vi "Teleop.vi"(10 "Match Info":T1={"Autonomous Elapsed Seconds"=0.0, "TeleOp Elapsed Seconds"=0.0, "Disabled Elapsed Seconds"=0.0, "Visited Autonomous"=FALSE, "Visited TeleOp"=FALSE, "Visited Disabled"=FALSE, "Autonomous Settings"={"Autonomous Style"=enum."Independent", "VI Refnum"=refnum}}, 11 "Call Context":T2) -> ()   [LabVIEW 2014]
doc: "This VI is called for each TeleOp packet received from the DS where the robot is not disabled. It is often used to read from the joysticks and update I/O or to update setpoints for timed control loops. It should complete and return within 20 milliseconds or it may miss DS packets."
uses:
  <vilib>/Rock Robotics/WPI/DriverStation/WPI_DriverStationDerivedRobotMode.ctl
  <vilib>/Rock Robotics/WPI/DriverStation/WPI_DriverStationMatch Info.ctl
  <vilib>/Rock Robotics/WPI/RobotDrive/WPI_RobotDriveGetSetRefNum.vi
  <vilib>/Rock Robotics/WPI/Joystick/WPI_JoystickGetSetRefNum.vi
  <vilib>/Rock Robotics/Network Tables/SD Write Boolean Array.vi
  <vilib>/Rock Robotics/Network Tables/SD Write Numeric Array.vi
  <vilib>/Rock Robotics/Network Tables/SD Read Boolean.vi
  <vilib>/Rock Robotics/Network Tables/SD Read Number.vi
  <vilib>/Rock Robotics/WPI/RobotDrive/WPI_RobotDriveMecanumDrive_Cartesian.vi
panel:
  out "Sample Slider 0":dbl(slide) scale=0.0..5.0
  out "Sample Boolean 1":bool
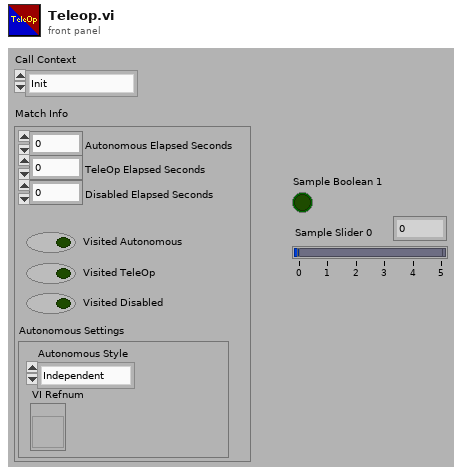
[diagram p1: front panel]
types:
  T1 = typedef "WPI_DriverStationMatch Info.ctl" = cluster{"Autonomous Elapsed Seconds":dbl, "TeleOp Elapsed Seconds":dbl, "Disabled Elapsed Seconds":dbl, "Visited Autonomous":bool, "Visited TeleOp":bool, "Visited Disabled":bool, "Autonomous Settings":cluster{"Autonomous Style":enum16{"Iterative", "Independent"}, "VI Refnum":refnum<vi>}}
  T2 = typedef "WPI_DriverStationDerivedRobotMode.ctl" = enum16{"Init", "Execute", "Stop"}
  T3 = typedef "WPI_JoystickDevRef.ctl" = cluster{"Device":T4}
  T4 = typedef "WPI_JoystickDeviceEnum.ctl" = enum16{"USB 0", "USB 1", "USB 2", "USB 3", "USB 4", "USB 5"}
  T5 = cluster{"Button 1":bool, "Button 2":bool, "Button 3":bool, "Button 4":bool, "Button 5":bool, "Button 6":bool, "Button 7":bool, "Button 8":bool, "Button 9":bool, "Button 10":bool, "Button 11":bool, "Button 12":bool}
  T6 = typedef "WPI_MotorControlDeviceRef.ctl" = cluster{"DeviceStatus":errorcluster, "Type":T7, "PWM":cluster{"Controller":T8, "PWM Channel":T9, "DeadBand":T10}, "CAN":cluster{"Device Number":u8, "Control Mode":T11, "Semaphore":T12, "Max Vout":dbl, "TalonSRX Control Mode":T13}, "Invert":bool, "TransformRef":T14, "InvTransformRef":T14}
  T7 = typedef "WPI_MotorControlType.ctl" = enum16{"PWM", "CAN", "CANTalonSRX"}
  T8 = typedef "FPGA_TypedefDigitalModule.ctl" = enum16{"Controller 1"}
  T9 = typedef "FPGA_DIOPWMChannel.ctl" = enum8{"PWM 0", "PWM 1", "PWM 2", "PWM 3", "PWM 4", "PWM 5", "PWM 6", "PWM 7", "PWM 8", "PWM 9", "PWM MXP 0", "PWM MXP 1", "PWM MXP 2", "PWM MXP 3", "PWM MXP 4", "PWM MXP 5", "PWM MXP 6", "PWM MXP 7", "PWM MXP 8", "PWM MXP 9", "Invalid"}
  T10 = typedef "WPI_PWMDeadband.ctl" = cluster{"Name":string, "maxPositivePwm":i32, "minPositivePwm":i32, "centerPwm":i32, "maxNegativePwm":i32, "minNegativePwm":i32, "angularRange":u16}
  T11 = typedef "WPI_CANJaguar_ControlMode.ctl" = enum8{"Percent VBus", "Current", "Speed", "Position", "Voltage"}
  T12 = typedef "Semaphore RefNum" = refnum<k1>
  T13 = typedef "WPI_CANTalonSRX_APIControlMode.ctl" = enum8{"Percent VBus", "Speed", "Position", "Slave", "Unchanged / Invalid"}
  T14 = typedef "WPI_PWMTransform_ConPane.ctl" = refnum<vi>
  T15 = typedef "WPI_RobotDriveDevRef.ctl" = cluster{"DevStatus":errorcluster, "Motors[]":T6[], "Square Inputs":bool, "Max Output":dbl}
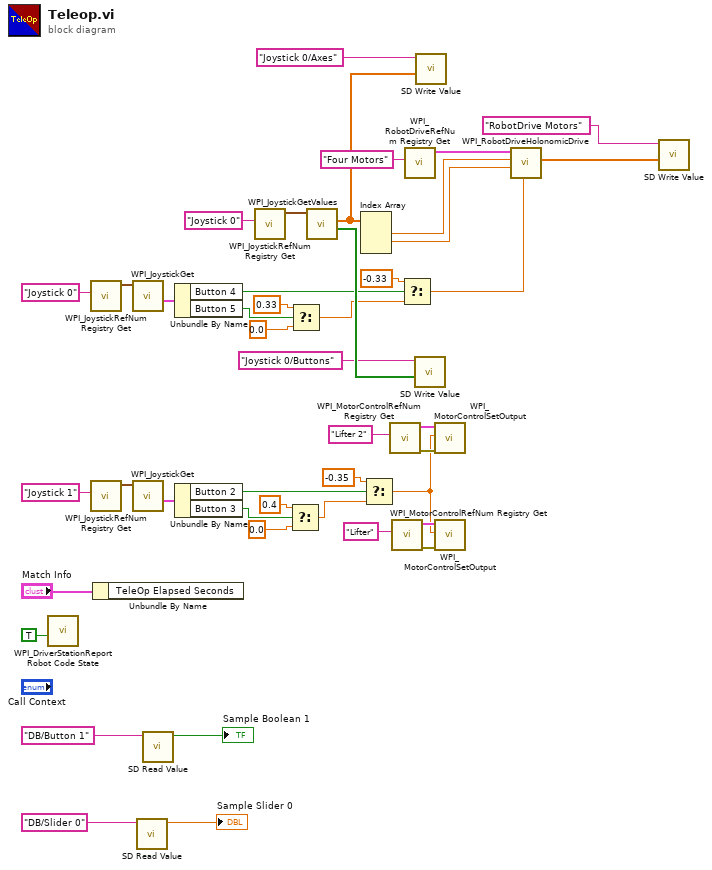
[diagram p0: block diagram]
diagram:
  n1 = call <vilib>:"WPI_DriverStationReport Robot Code State.vi"("TeleOp"=TRUE ("Autonomous")) -> ()  [unwired: 10 in, 1 out]
  n2 = call <vilib>:"WPI_JoystickRefNum Registry Get.vi"("refnum name"="Joystick 0") -> ("JoystickDevRef"=w25:T3)  [unwired: 1 in, 9 out]
  n3 = call <vilib>:"WPI_JoystickRefNum Registry Get.vi"("refnum name"="Joystick 1") -> ("JoystickDevRef"=w17:T3)  [unwired: 1 in, 9 out]
  n4 = Unbundle By Name("Match Info") -> ()  [unwired: 1 out]
  n5 = call <vilib>:"WPI_JoystickGet.vi"("JoystickDevRef"=w25) -> ("Buttons"=w26:T5)  [unwired: 1 in, 5 out]
  n6 = call <vilib>:"WPI_JoystickGet.vi"("JoystickDevRef"=w17) -> ("Buttons"=w18:T5)  [unwired: 1 in, 5 out]
  n7 = call-poly <vilib>:"SD Read Value.vi"("Name"="DB/Slider 0" ("refnum name")) -> ("Numeric"=→"Sample Slider 0":dbl)  [unwired: 8 in, 2 out]
  n8 = call-poly <vilib>:"SD Read Value.vi"("Name"="DB/Button 1" ("refnum name")) -> ("Boolean"=→"Sample Boolean 1":bool)  [unwired: 8 in, 2 out]
  n9 = Unbundle By Name(w26) -> ("Button 4"=w22:bool, "Button 5"=w21:bool)
  n10 = Unbundle By Name(w18) -> ("Button 2"=w15:bool, "Button 3"=w14:bool)
  n11 = call <vilib>:"WPI_JoystickRefNum Registry Get.vi"("refnum name"="Joystick 0") -> ("JoystickDevRef"=w39:T3)  [unwired: 1 in, 9 out]
  n12 = Select(t=0.4, s=w14, f=0.0) -> (s? t:f=w2:dbl)
  n13 = Select(t=0.33, s=w21, f=0.0) -> (s? t:f=w3:dbl)
  n14 = call <vilib>:"WPI_JoystickGetValues.vi"("JoystickDevRef"=w39) -> ("Buttons"=w37:bool[], "Axes"=w27:dbl[])  [unwired: 6 in, 3 out]
  n15 = Index Array "Index Array"(array=w27) -> (element #1=w41:dbl, element #2=w29:dbl)  [unwired: 3 in, 1 out]
  n16 = Select(t=-0.35 ("x"), s=w15, f=w2) -> (s? t:f=w1:dbl)
  n17 = call <vilib>:"WPI_MotorControlRefNum Registry Get.vi"("refnum name"="Lifter 2") -> ("error out"=w10:errorcluster, "MotorControlDevRef"=w8:T6)  [unwired: 9 in]
  n18 = call <vilib>:"WPI_MotorControlRefNum Registry Get.vi"("refnum name"="Lifter") -> ("error out"=w13:errorcluster, "MotorControlDevRef"=w11:T6)  [unwired: 9 in]
  n19 = Select(t=-0.33, s=w22, f=w3) -> (s? t:f=w4:dbl)
  n20 = call <vilib>:"WPI_RobotDriveRefNum Registry Get.vi"("refnum name"="Four Motors") -> ("RobotDriveDevRef"=w42:T15)  [unwired: 1 in, 9 out]
  n21 = call-poly <vilib>:"SD Write Value.vi"("Boolean Array"=w37, "Name"="Joystick 0/Buttons") -> ()  [unwired: 8 in, 2 out]
  n22 = call-poly <vilib>:"SD Write Value.vi"("Numeric Array"=w27, "Name"="Joystick 0/Axes") -> ()  [unwired: 8 in, 2 out]
  n23 = call <vilib>:"WPI_MotorControlSetOutput.vi"("error in (no error)"=w10, "Output"=w1, "MotorControlDevRef"=w8) -> ()  [unwired: 6 in, 3 out]
  n24 = call <vilib>:"WPI_MotorControlSetOutput.vi"("error in (no error)"=w13, "Output"=w1, "MotorControlDevRef"=w11) -> ()  [unwired: 6 in, 3 out]
  n25 = call-poly <vilib>:"WPI_RobotDriveHolonomicDrive.vi"("Rotation"=w4, "Y"=w29, "X"=w41, "RobotDriveDevRef"=w42) -> ("Motor Values"=w28:dbl[])  [unwired: 5 in, 2 out]
  n26 = call-poly <vilib>:"SD Write Value.vi"("Numeric Array"=w28, "Name"="RobotDrive Motors") -> ()  [unwired: 8 in, 2 out]
